vi "Save-Recall Setup.vi"(8 "error in (no error)":errorcluster, 9 "Pannel Setup (1)":i8=1, 10 "Mode (T:Save)":bool=TRUE, 11 "VISA resource name":refnum<visa-resource-name>) -> (0 "error out":errorcluster, 3 "VISA resource name out":refnum<visa-resource-name>)   [LabVIEW 2015, in "LeCroy Wave Series.lvlib"]
doc: "Stores/Recall the current state of your instrument in/from non-volatile internal memory. Stores the complete front panel setup of the oscilloscope at the time the command is issued, or setup front panel from non-volatile internal memory."
uses:
  <instrlib>/LeCroy Wave Series/LeCroy Wave Series.lvlib
panel:
  # "Save\n\nRecall"
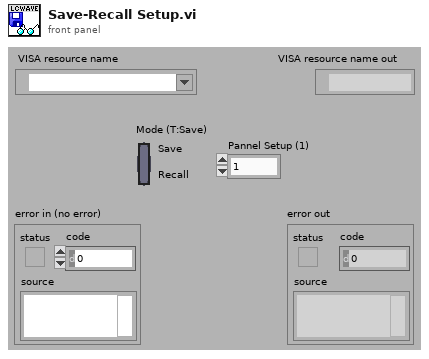
[diagram p1: front panel]
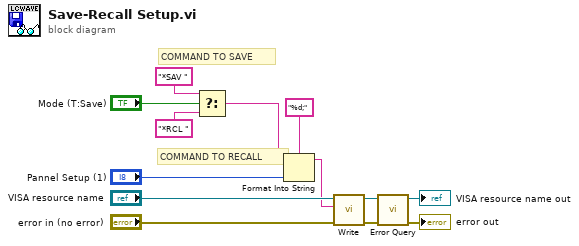
[diagram p0: block diagram]
diagram:
  # "COMMAND TO RECALL"
  # "COMMAND TO SAVE"
  n1 = Select(t="*SAV ", s="Mode (T:Save)", f="*RCL ") -> (s? t:f=w2:string)
  n2 = Format Into String(format string="%d;", initial string=w2, "Pannel Setup (1)") -> (resulting string=w1:string)  [unwired: 1 in, 1 out]
  n3 = call <instrlib>:"Write.vi"("error in (no error)"="error in (no error)", "Write Buffer"=w1, "VISA resource name"="VISA resource name") -> ("error out"=w8:errorcluster, "VISA resource name out"=w9:refnum<visa-resource-name>)  [unwired: 6 in, 1 out]
  n4 = call <instrlib>:"Error Query.vi"("error in (no error)"=w8, "VISA resource name"=w9) -> ("error out"=→"error out":errorcluster, "VISA resource name out"=→"VISA resource name out":refnum<visa-resource-name>)  [unwired: 6 in, 2 out]
